vi "Abs_Current_Time.vi"() -> (1 "Abs_Time.lvclass":refnum<class "Abs_Time.lvclass">)   [LabVIEW 2021]
uses:
  Abs_Types/Time/Abs_Time.lvclass
  Support/Curr_Time/Const_Current Time.lvclass
  C:/Program Files (x86)/National Instruments/LabVIEW 2021/vi.lib/TSA/Abstract Data Classes/Abs_Types/Time/Abs_Time.lvclass
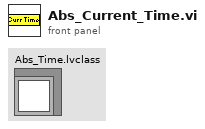
[diagram p1: front panel]
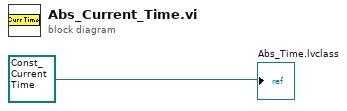
[diagram p0: block diagram]
diagram:
  "Abs_Time.lvclass" <- refnum<class "Const_Current Time.lvclass"> refnum ("Const_Current Time.lvclass")
